vi "HwManager.vi"(6 "InstrumentHandle_port in":u32, 7 "action (Init)":T2, 8 "error in (no error)":errorcluster, 9 "InstrumentHandle_board in":u32, 10 "port":u32, 11 "board":u32) -> (0 "error out":errorcluster, 1 "validityFlag":T1, 2 "InstrumentHandle_port out":u32, 3 "InstrumentHandle_board out":u32, 4 "Duplicated":bool)   [LabVIEW 2020, in "AIM664LV.lvlib"]
uses:
  AIM664LV.lvlib
  _controls/hwEntry_actions.ctl
  _controls/hwEntry_handleValidityFlag.ctl
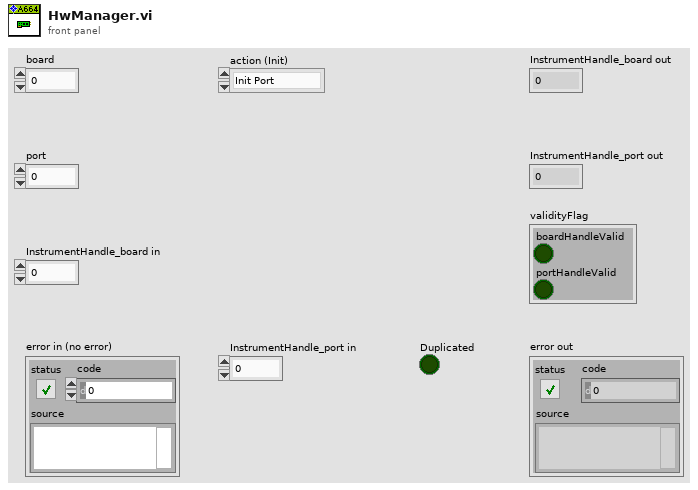
[diagram p1: front panel]
types:
  T1 = typedef "AIM664LV.lvlib/hwEntry_handleValidityFlag.ctl" = cluster{"boardHandleValid":bool, "portHandleValid":bool}
  T2 = typedef "AIM664LV.lvlib/hwEntry_actions.ctl" = enum16{"Init Port", "Init Board", "Relase Port", "Release Board"}
  T3 = typedef "AIM664LV.lvlib/hwEntryBoardResource.ctl" = cluster{"InstrumentHandle_board":u32, "boardresource":cluster{"ResourceID":u32, "ResourceType":u32, "ResourceInfo":string, "StructId":u32}, "Ports":map{u32, T4}}
  T4 = typedef "AIM664LV.lvlib/hwEntryPortResource.ctl" = cluster{"InstrumentHandle_port":u32, "boardresource":cluster{"ResourceID":u32, "ResourceType":u32, "ResourceInfo":string, "StructId":u32}}
  T5 = typedef "AIM664LV.lvlib/hwEntry_data.ctl" = cluster{"handleMap":map{u32, T6}, "resourceMap":map{u32, T3}}
  T6 = typedef "AIM664LV.lvlib/hwEntryBoardHandleMap.ctl" = cluster{"boardId":u32, "portHandleMap":map{u32, u32}}
  T7 = cluster{"ResourceID":u32, "ResourceType":u32, "ResourceInfo":string, "StructId":u32}
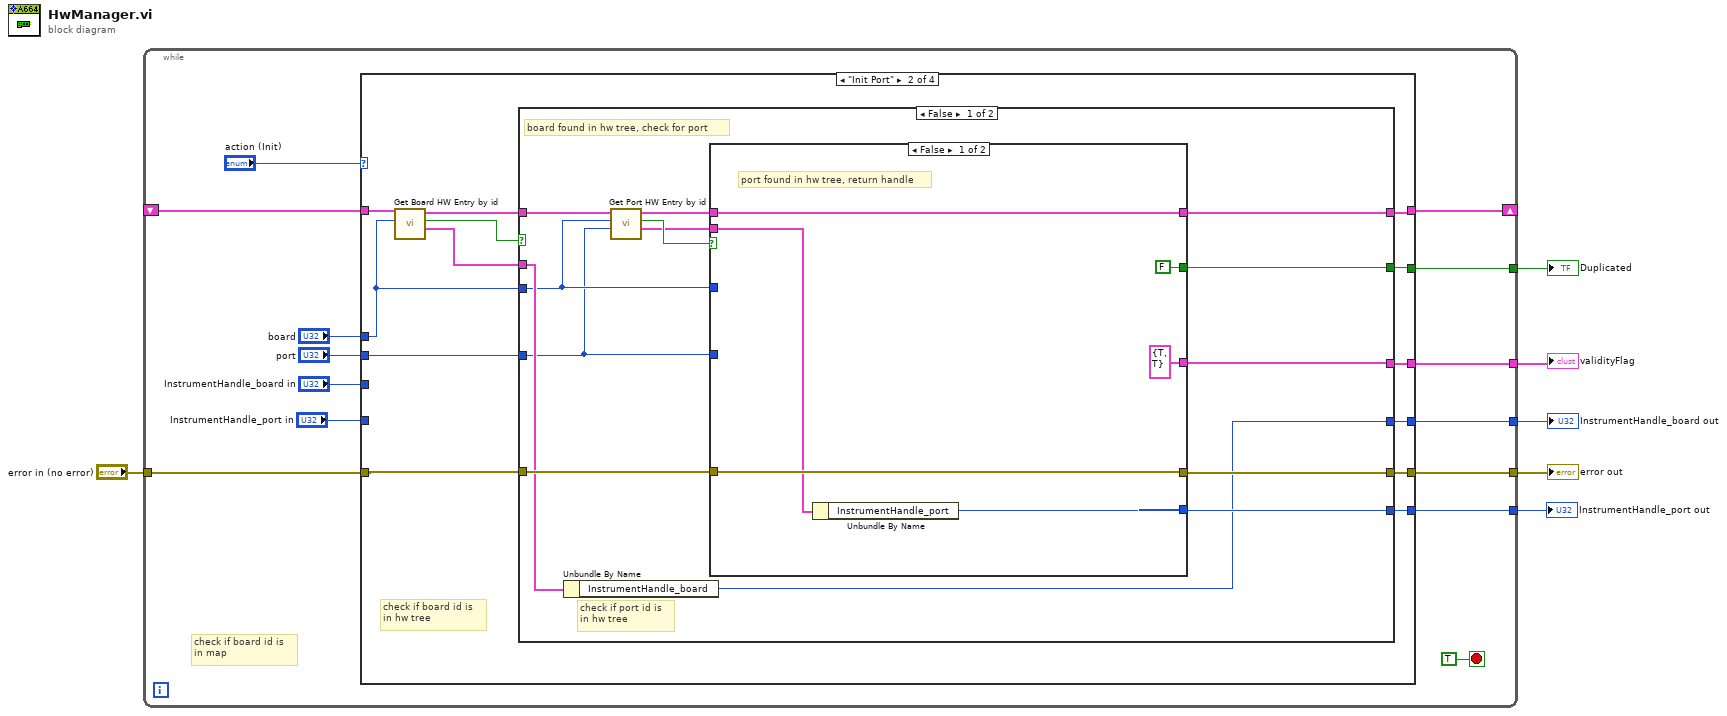
[diagram p0: block diagram]
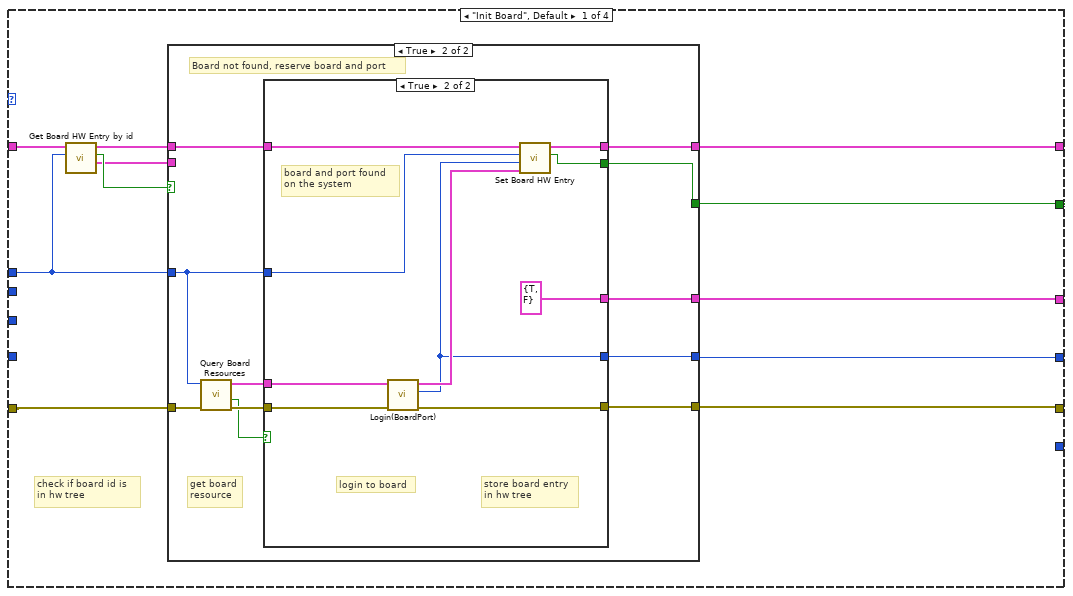
[diagram p2: hidden frame]
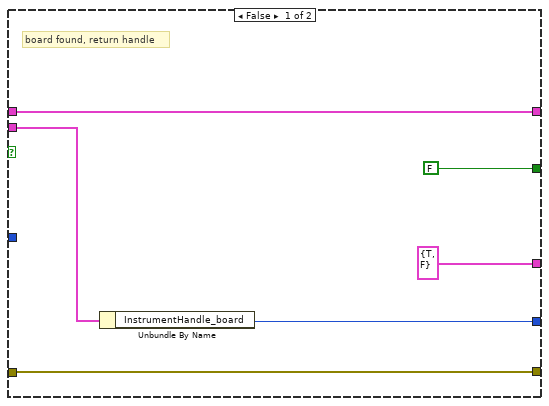
[diagram p3: hidden frame]
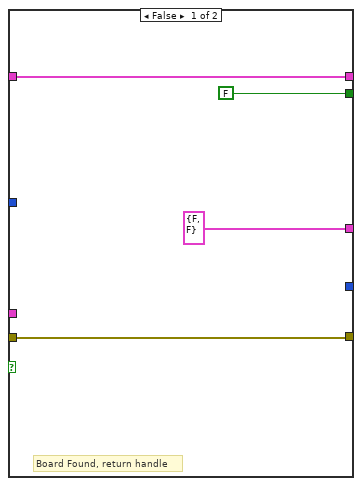
[diagram p4: hidden frame]
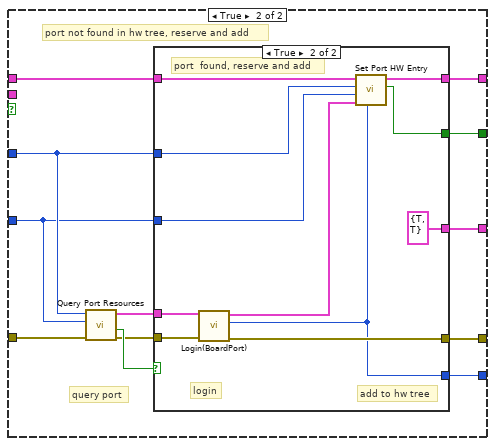
[diagram p5: hidden frame]
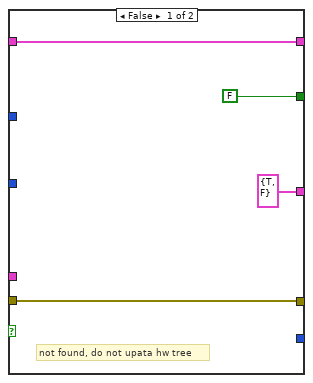
[diagram p6: hidden frame]
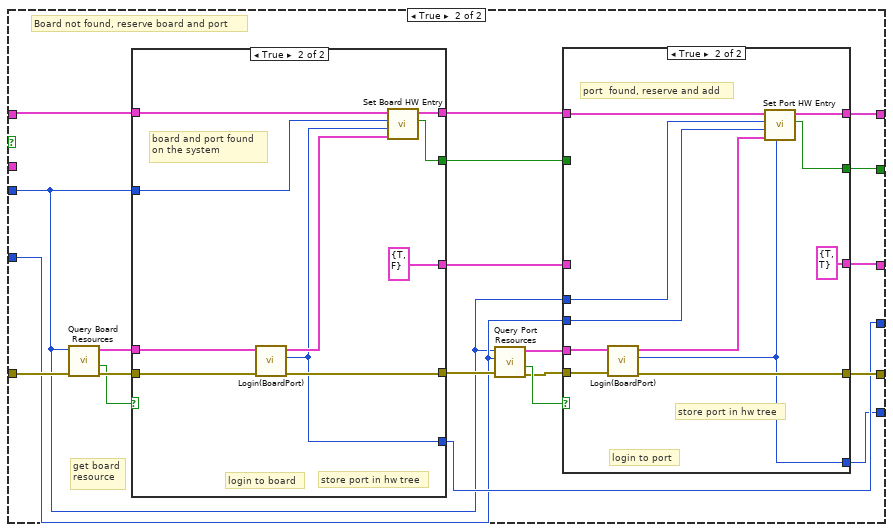
[diagram p7: hidden frame]
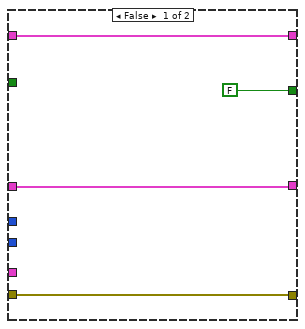
[diagram p8: hidden frame]
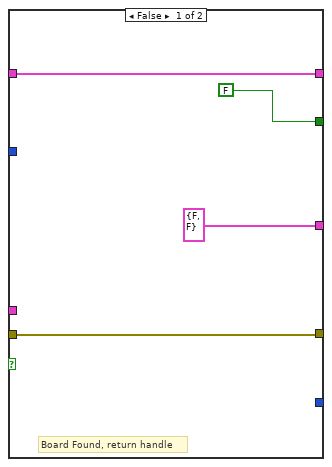
[diagram p9: hidden frame]
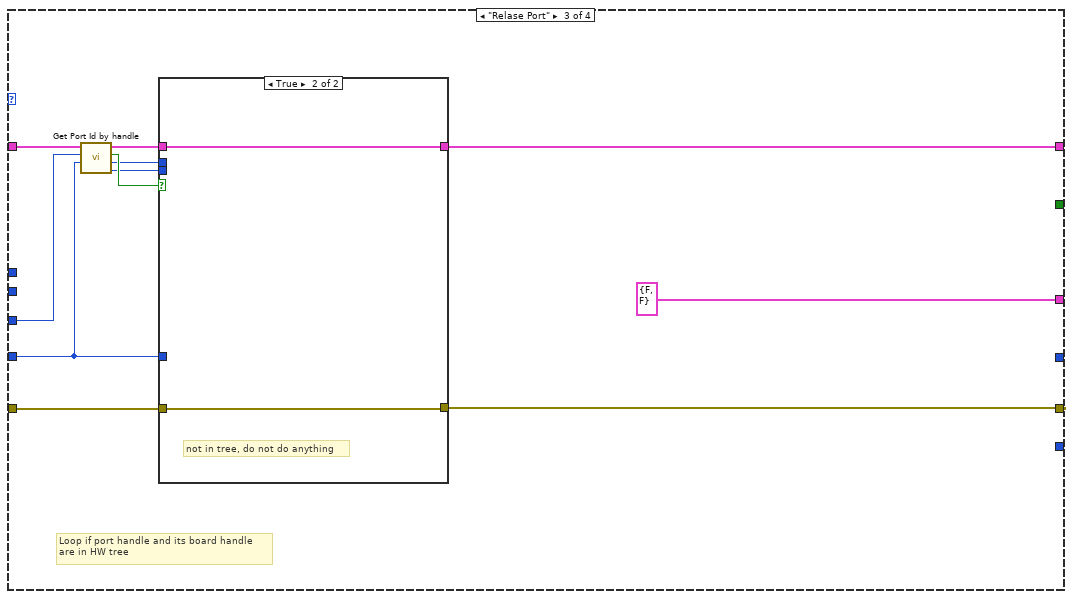
[diagram p10: hidden frame]
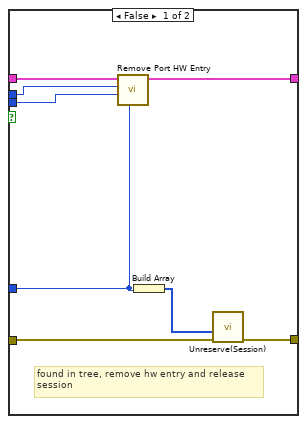
[diagram p11: hidden frame]
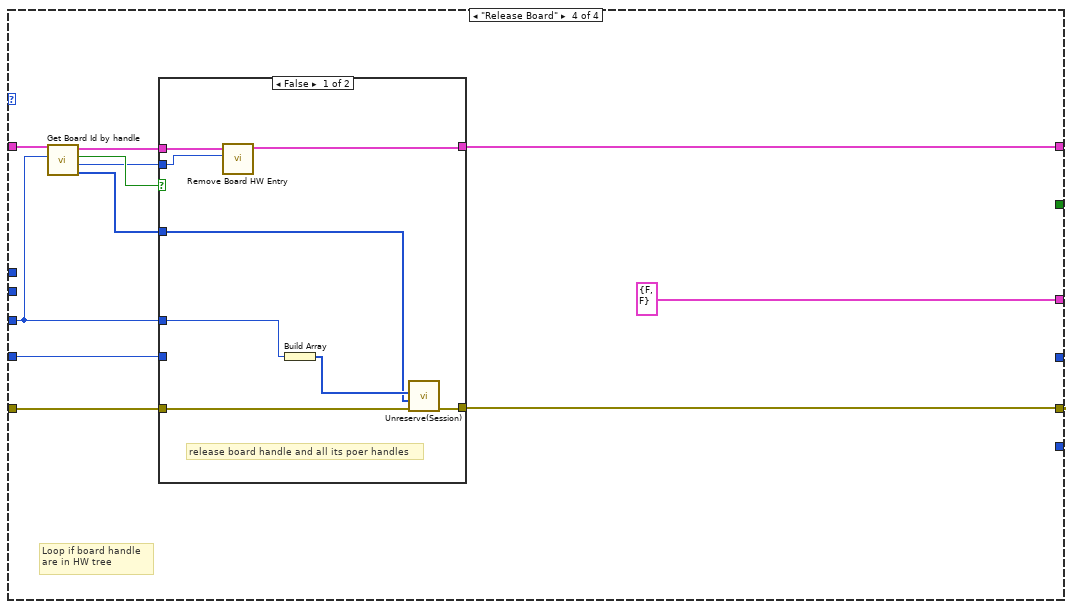
[diagram p12: hidden frame]
diagram:
  n1 = while {
    tunnel: "error in (no error)" -> [w18]
    tunnel: [w15] -> w5
    tunnel: [w14] -> w4
    tunnel: [w11] -> w2
    tunnel: [w10] -> w3
    tunnel: [w9] -> w1
    shift-right: [w7] -> _
    shift-left: _ -> [w8]
    stop <- TRUE stop-if-true
    # "check if board id is \nin map"
    n2 = case shown="\"Init Port\"" "action (Init)" {
      tunnel: w18 -> [w31 w75 w181 w202]
      tunnel: "board" -> [w24 w64 _ _]
      tunnel: "port" -> [_ w73 _ _]
      tunnel: [w29 w71 _ _] -> w15
      tunnel: [w28 w72 w175 w200] -> w14
      tunnel: "InstrumentHandle_board in" -> [_ _ w177 w194]
      tunnel: "InstrumentHandle_port in" -> [_ _ w176 w201]
      tunnel: [w27 w70 T1 {"boardHandleValid"=FALSE, "portHandleValid"=FALSE} ("validityFlag") T1 {"boardHandleValid"=FALSE, "portHandleValid"=FALSE} ("validityFlag")] -> w11
      tunnel: [w26 w74 _ _] -> w10
      tunnel: [w30 w63 w174 w199] -> w7
      tunnel: [_ w69 _ _] -> w9
      tunnel: w8 -> [w25 w68 w180 w198]
      frame "Init Board", Default {
        # "check if board id is \nin hw tree"
        n3 = call "Get Board HW Entry by id.vi"("board"=w24, "hw_data in"=w25) -> ("board resource out"=w21:T3, "key not found?"=w22:bool, "hw_data out"=w23:T5)  [unwired: 7 in]
        n4 = case shown="True" w22 {
          tunnel: w31 -> [w35 w48]
          tunnel: [w35 w44] -> w28
          tunnel: [w32 w42] -> w29
          tunnel: [T1 {"boardHandleValid"=TRUE, "portHandleValid"=FALSE} ("validityFlag") w43] -> w27
          tunnel: [FALSE ("key already included?") w40] -> w26
          tunnel: w24 -> [_ w39]
          tunnel: [w34 w41] -> w30
          tunnel: w23 -> [w34 w38]
          tunnel: w21 -> [w33 _]
          frame False {
            # "board found, return handle"
            n5 = Unbundle By Name(w33) -> ("InstrumentHandle_board"=w32:u32)
          }
          frame True {
            # "get board\nresource"
            # "Board not found, reserve board and port"
            n6 = call "Query Board Resources.vi"("error in (no error)"=w48, "board"=w39) -> ("error out"=w46:errorcluster, "found"=w45:bool, "board resource"=w47:T7)  [unwired: 7 in]
            n7 = case shown="True" w45 {
              tunnel: w47 -> [_ w61]
              tunnel: w46 -> [w52 w62]
              tunnel: [w52 w60] -> w44
              tunnel: [T1 {"boardHandleValid"=FALSE, "portHandleValid"=FALSE} ("validityFlag") T1 {"boardHandleValid"=TRUE, "portHandleValid"=FALSE} ("validityFlag")] -> w43
              tunnel: [_ w55] -> w42
              tunnel: [w49 w57] -> w41
              tunnel: [FALSE ("key already included?") w53] -> w40
              tunnel: w39 -> [_ w54]
              tunnel: w38 -> [w49 w58]
              frame False {
                # "Board Found, return handle"
              }
              frame True {
                # "store board entry \nin hw tree"
                # "login to board"
                # "board and port found\non the system"
                n8 = call "Login(BoardPort).vi"("error in (no error)"=w62, "resource in"=w61) -> ("error out"=w60:errorcluster, "Handle"=w55:u32, "resource out"=w56:T7)  [unwired: 7 in]
                n9 = call "Set Board HW Entry.vi"("boardresource"=w56, "InstrumentHandle_board"=w55, "boardId"=w54, "hw_data in"=w58) -> ("duplicated"=w53:bool, "hw_data out"=w57:T5)  [unwired: 6 in]
              }
            }
          }
        }
      }
      frame "Init Port" {
        # "check if board id is \nin hw tree"
        n10 = call "Get Board HW Entry by id.vi"("board"=w64, "hw_data in"=w68) -> ("board resource out"=w65:T3, "key not found?"=w67:bool, "hw_data out"=w66:T5)  [unwired: 7 in]
        n11 = case shown="False" w67 {
          tunnel: w75 -> [w89 w138]
          tunnel: [w86 w132] -> w74
          tunnel: w73 -> [w79 w125]
          tunnel: [w88 w131] -> w72
          tunnel: [w82 w130] -> w71
          tunnel: [w85 w134] -> w70
          tunnel: [w84 w129] -> w69
          tunnel: w66 -> [w81 w139]
          tunnel: w65 -> [w83 _]
          tunnel: w64 -> [w80 w124]
          tunnel: [w87 w133] -> w63
          frame False {
            # "check if port id is \nin hw tree"
            # "board found in hw tree, check for port"
            n12 = Unbundle By Name(w83) -> ("InstrumentHandle_board"=w82:u32)
            n13 = call "Get Port HW Entry by id.vi"("port"=w79, "board"=w80, "hw_data in"=w81) -> ("port hw entry out"=w76:T4, "key not found?"=w77:bool, "hw_data out"=w78:T5)  [unwired: 6 in]
            n14 = case shown="False" w77 {
              tunnel: w78 -> [w94 w105]
              tunnel: w89 -> [w95 w107]
              tunnel: w80 -> [_ w104]
              tunnel: w79 -> [_ w103]
              tunnel: [w95 w101] -> w88
              tunnel: [w94 w100] -> w87
              tunnel: [FALSE ("duplicated") w99] -> w86
              tunnel: [T1 {"boardHandleValid"=TRUE, "portHandleValid"=TRUE} ("validityFlag") w98] -> w85
              tunnel: [w90 w97] -> w84
              tunnel: w76 -> [w91 _]
              frame False {
                # "port found in hw tree, return handle"
                n15 = Unbundle By Name(w91) -> ("InstrumentHandle_port"=w90:u32)
              }
              frame True {
                # "query port"
                # "port not found in hw tree, reserve and add"
                n16 = call "Query Port Resources.vi"("error in (no error)"=w107, "port"=w103, "board"=w104) -> ("error out"=w102:errorcluster, "found"=w106:bool, "port resource"=w96:T7)  [unwired: 6 in]
                n17 = case shown="True" w106 {
                  tunnel: w105 -> [w111 w122]
                  tunnel: w104 -> [_ w121]
                  tunnel: w103 -> [_ w120]
                  tunnel: w102 -> [w108 w119]
                  tunnel: [w108 w117] -> w101
                  tunnel: [w111 w116] -> w100
                  tunnel: [FALSE ("duplicated") w115] -> w99
                  tunnel: [T1 {"boardHandleValid"=TRUE, "portHandleValid"=FALSE} ("validityFlag") T1 {"boardHandleValid"=TRUE, "portHandleValid"=TRUE} ("validityFlag")] -> w98
                  tunnel: [_ w114] -> w97
                  tunnel: w96 -> [_ w112]
                  frame False {
                    # "not found, do not upata hw tree"
                  }
                  frame True {
                    # "add to hw tree"
                    # "login"
                    # "port  found, reserve and add"
                    n18 = call "Login(BoardPort).vi"("error in (no error)"=w119, "resource in"=w112) -> ("error out"=w117:errorcluster, "Handle"=w114:u32, "resource out"=w118:T7)  [unwired: 7 in]
                    n19 = call "Set Port HW Entry.vi"("InstrumentHandle_port"=w114, "boardresource"=w118, "portId"=w120, "boardId"=w121, "hw_data in"=w122) -> ("duplicated"=w115:bool, "hw_data out"=w116:T5)  [unwired: 5 in]
                  }
                }
              }
            }
          }
          frame True {
            # "get board\nresource"
            # "Board not found, reserve board and port"
            n20 = call "Query Board Resources.vi"("error in (no error)"=w138, "board"=w124) -> ("error out"=w141:errorcluster, "found"=w140:bool, "board resource"=w142:T7)  [unwired: 7 in]
            n21 = case shown="True" w140 {
              tunnel: w142 -> [_ w170]
              tunnel: w141 -> [w161 w171]
              tunnel: [w161 w169] -> w127
              tunnel: [T1 {"boardHandleValid"=FALSE, "portHandleValid"=FALSE} ("validityFlag") T1 {"boardHandleValid"=TRUE, "portHandleValid"=FALSE} ("validityFlag")] -> w128
              tunnel: [_ w164] -> w130
              tunnel: [w158 w166] -> w135
              tunnel: [FALSE ("key already included?") w163] -> w123
              tunnel: w139 -> [w158 w167]
              tunnel: w124 -> [_ w162]
              frame False {
                # "Board Found, return handle"
              }
              frame True {
                # "store port in hw tree"
                # "login to board"
                # "board and port found\non the system"
                n22 = call "Login(BoardPort).vi"("error in (no error)"=w171, "resource in"=w170) -> ("error out"=w169:errorcluster, "Handle"=w164:u32, "resource out"=w165:T7)  [unwired: 7 in]
                n23 = call "Set Board HW Entry.vi"("boardresource"=w165, "InstrumentHandle_board"=w164, "boardId"=w162, "hw_data in"=w167) -> ("duplicated"=w163:bool, "hw_data out"=w166:T5)  [unwired: 6 in]
              }
            }
            n24 = call "Query Port Resources.vi"("error in (no error)"=w127, "port"=w125, "board"=w124) -> ("error out"=w136:errorcluster, "found"=w137:bool, "port resource"=w126:T7)  [unwired: 6 in]
            n25 = case shown="True" w137 {
              tunnel: w135 -> [w146 w157]
              tunnel: w136 -> [w144 w156]
              tunnel: [w144 w154] -> w131
              tunnel: [w146 w153] -> w133
              tunnel: [FALSE ("duplicated") w152] -> w132
              tunnel: [w143 T1 {"boardHandleValid"=TRUE, "portHandleValid"=TRUE} ("validityFlag")] -> w134
              tunnel: [_ w151] -> w129
              tunnel: w128 -> [w143 _]
              tunnel: w126 -> [_ w149]
              tunnel: w124 -> [_ w148]
              tunnel: w125 -> [_ w147]
              tunnel: w123 -> [_ _]
              frame False {
              }
              frame True {
                # "store port in hw tree"
                # "login to port"
                # "port  found, reserve and add"
                n26 = call "Login(BoardPort).vi"("error in (no error)"=w156, "resource in"=w149) -> ("error out"=w154:errorcluster, "Handle"=w151:u32, "resource out"=w155:T7)  [unwired: 7 in]
                n27 = call "Set Port HW Entry.vi"("InstrumentHandle_port"=w151, "boardresource"=w155, "portId"=w147, "boardId"=w148, "hw_data in"=w157) -> ("duplicated"=w152:bool, "hw_data out"=w153:T5)  [unwired: 5 in]
              }
            }
          }
        }
      }
      frame "Relase Port" {
        # "Loop if port handle and its board handle\nare in HW tree"
        n28 = call "Get Port Id by handle.vi"("port handle"=w176, "board handle"=w177, "hw_data in"=w180) -> ("portId"=w172:u32, "boardId"=w173:u32, "key not found?"=w178:bool, "hw_data out"=w179:T5)  [unwired: 5 in]
        n29 = case shown="True" w178 {
          tunnel: w181 -> [w189 w192]
          tunnel: w179 -> [w187 w191]
          tunnel: w176 -> [w183 _]
          tunnel: [w188 w192] -> w175
          tunnel: [w186 w191] -> w174
          tunnel: w173 -> [w185 _]
          tunnel: w172 -> [w184 _]
          frame False {
            # "found in tree, remove hw entry and release\nsession"
            n30 = call "Remove Port HW Entry.vi"("InstrumentHandle_port"=w183, "portId"=w184, "boardId"=w185, "hw_data in"=w187) -> ("hw_data out"=w186:T5)  [unwired: 7 in]
            n31 = Build Array(w183) -> (w190:u32[])
            n32 = call "Unreserve(Session).vi"("error in (no error)"=w189, "InstrumentHandle_port in"=w190) -> ("error out"=w188:errorcluster)  [unwired: 9 in]
          }
          frame True {
            # "not in tree, do not do anything"
          }
        }
      }
      frame "Release Board" {
        # "Loop if board handle\nare in HW tree"
        n33 = call "Get Board Id by handle.vi"("board handle"=w194, "hw_data in"=w198) -> ("port handles"=w193:u32[], "boardId"=w195:u32, "key not found"=w197:bool, "hw_data out"=w196:T5)  [unwired: 6 in]
        n34 = case shown="False" w197 {
          tunnel: w202 -> [w211 w213]
          tunnel: w201 -> [_ _]
          tunnel: [w210 w213] -> w200
          tunnel: [w205 w212] -> w199
          tunnel: w196 -> [w206 w212]
          tunnel: w195 -> [w204 _]
          tunnel: w194 -> [w209 _]
          tunnel: w193 -> [w207 _]
          frame False {
            # "release board handle and all its poer handles"
            n35 = call "Remove Board HW Entry.vi"("boardId"=w204, "hw_data in"=w206) -> ("hw_data out"=w205:T5)  [unwired: 9 in]
            n36 = Build Array(w209) -> (w208:u32[])
            n37 = call "Unreserve(Session).vi"("error in (no error)"=w211, "InstrumentHandle_port in"=w207, "InstrumentHandle_board in"=w208) -> ("error out"=w210:errorcluster)  [unwired: 8 in]
          }
          frame True {
          }
        }
      }
    }
  }
  "validityFlag" <- w2
  "InstrumentHandle_port out" <- w1
  "InstrumentHandle_board out" <- w5
  "error out" <- w4
  "Duplicated" <- w3
